vi "PROYECTO.vi"() -> ()   [LabVIEW 2021]
uses:
  <vilib>/userDefined/High Color/IMAQdx.ctl
  <vilib>/addons/database/Connection.llb/DB Tools Open Connec (Path).vi
  <vilib>/Instr/_visa.llb/VISA Configure Serial Port (Instr).vi
  <vilib>/addons/database/Connection.llb/Conn Execute.vi
  <vilib>/addons/database/Recordset.llb/Rec Fetch String Data (R).vi
  <vilib>/addons/database/Recordset.llb/Rec Destroy - Connection.vi
  <vilib>/vision/driver/NI_Vision_Acquisition_Software.lvlib
  <vilib>/vision/NI_Vision_Development_Module.lvlib
  <vilib>/addons/database/NI_Database_API.lvlib
panel:
  in  "VISA resource name":refnum<visa-resource-name>
  in  "connection information":path
  out "Placa Encontrada":string
  out "Consulta":string
  out "Read String":string
  in  "Rectangle":T1 {"Rotation" min=-90.0 max=90.0 step=1.0 format="%.2f"; "Left" scale=0.0..1024.0; "Right" scale=0.0..1024.0}
  out "Image":T2(plugin-control)
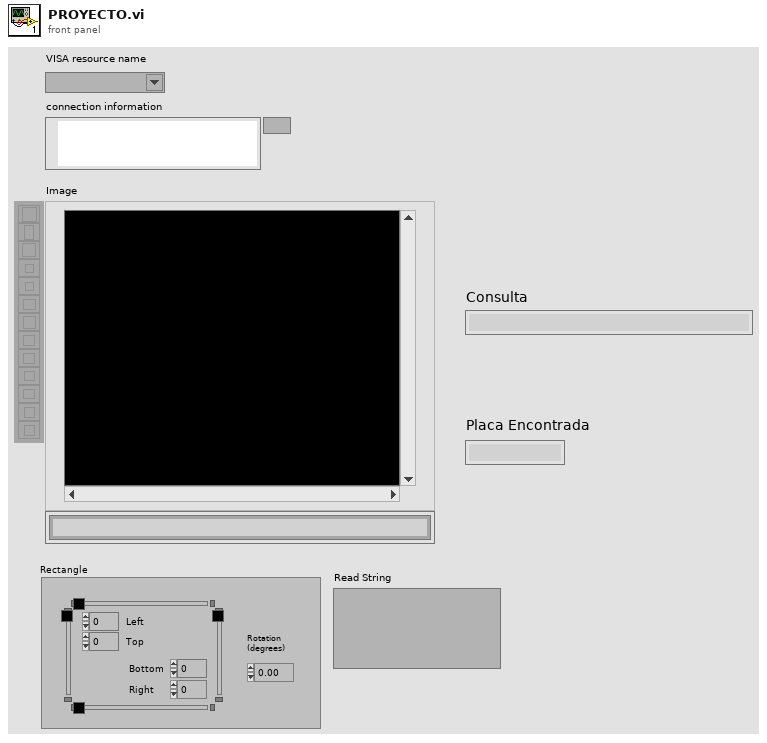
[diagram p1: front panel]
types:
  T1 = typedef "IMAQ Rectangle" = cluster{"Left":i32, "Top":i32, "Right":i32, "Bottom":i32, "Rotation":dbl}
  T2 = typedef "IMAQ Image.ctl" = refnum<image>
  T3 = typedef "IMAQdx.ctl" = refnum<k21>
  T4 = typedef "IMAQ OCR Session.ctl" = refnum<k1>
  T5 = typedef "ROI Descriptor" = cluster{"Global Rectangle":i32[], "Contours":cluster{"ID":enum32{"External", "Internal"}, "Type":u32, "Coordinates":i32[]}[]}
  T6 = typedef "NI_Database_API.lvlib/Conn ObjectReference.ctl" = refnum<k1>
  T7 = cluster{"Global Rectangle":i32[], "Contours":cluster{"ID":enum32{"External", "Internal"}, "Type":u32, "Coordinates":i32[]}[]}
  T8 = typedef "NI_Database_API.lvlib/Rec ObjectReference.ctl" = refnum<k1>
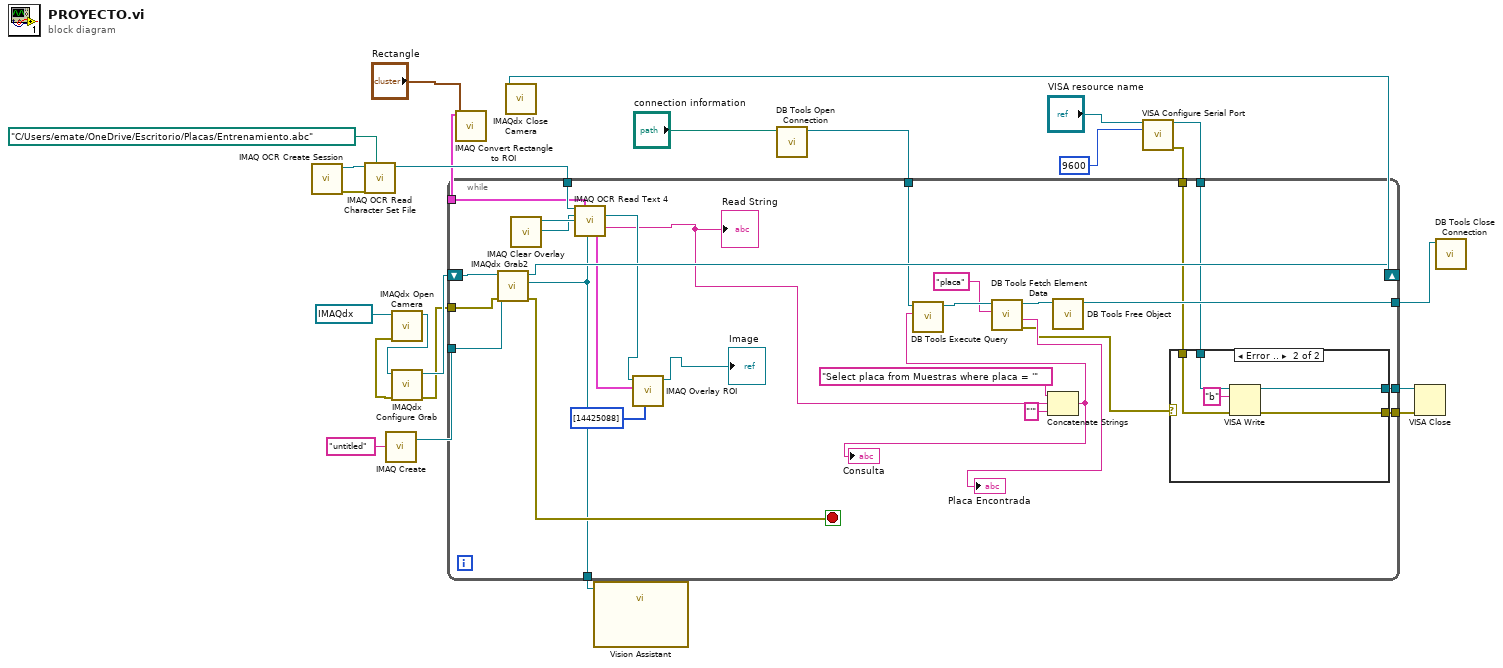
[diagram p0: block diagram]
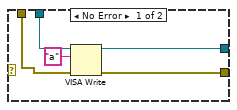
[diagram p2: hidden frame]
diagram:
  n1 = call "IMAQ OCR Create Session"() -> ("error out"=w15:errorcluster, "IMAQ OCR Session"=w16:T4)  [unwired: 10 in]
  n2 = call "IMAQ OCR Read Character Set File"("File Path"=path "C:/Users/emate/OneDrive/Escritorio/Placas/Entrenamiento.abc", "error in (no error)"=w15, "IMAQ OCR Session"=w16) -> ("IMAQ OCR Session (dup)"=w13:T4)  [unwired: 6 in, 2 out]
  n3 = call "IMAQ Create"("Image Name"="untitled") -> ("New Image"=w20:T2)  [unwired: 4 in, 1 out]
  n4 = call <vilib>:"IMAQdx Open Camera.vi"("Session In"=T3 "cam0") -> ("error out"=w23:errorcluster, "Session Out"=w24:T3)  [unwired: 9 in]
  n5 = call <vilib>:"IMAQdx Configure Grab.vi"("error in"=w23, "Session In"=w24) -> ("error out"=w19:errorcluster, "Session Out"=w22:T3)  [unwired: 8 in]
  n6 = call "IMAQ Convert Rectangle to ROI"("Rectangle"="Rectangle") -> ("ROI Descriptor"=w11:T5)  [unwired: 8 in, 1 out]
  n7 = call-poly <vilib>:"DB Tools Open Connection.vi"("connection information"="connection information") -> ("connection reference"=w8:T6)  [unwired: 7 in, 1 out]
  n8 = call-poly "VISA Configure Serial Port"("VISA resource name"="VISA resource name", "baud rate (9600)"=u32 9600) -> ("VISA resource name out"=w4:refnum<visa-resource-name>, "error out"=w3:errorcluster)  [unwired: 12 in]
  n9 = while {
    tunnel: w20 -> [w51]
    tunnel: w19 -> [w50]
    shift-right: [w49] -> w18
    shift-left: w22 -> [w52]
    tunnel: w13 -> [w48]
    tunnel: w11 -> [w47]
    tunnel: [w41] -> w10
    tunnel: w8 -> [w34]
    tunnel: [w29] -> w7
    tunnel: w4 -> [w28]
    tunnel: w3 -> [w27]
    tunnel: [w25] -> w2
    tunnel: [w26] -> w1
    stop <- w46 stop-if-true
    n10 = call <vilib>:"IMAQdx Grab2.vi"("error in"=w50, "Image In"=w51, "Session In"=w52) -> ("error out"=w46:errorcluster, "Image Out"=w41:T2, "Session Out"=w49:T3)  [unwired: 5 in, 1 out]
    n11 = call "IMAQ Clear Overlay"("Image"=w41) -> ("Image Out"=w40:T2)  [unwired: 9 in, 1 out]
    n12 = call "IMAQ OCR Read Text 4"("IMAQ OCR Session"=w48, "ROI Descriptor"=w47, "Image"=w40) -> ("Image (dup)"=w44:T2, "Read String"=w37:string, "ROI Bounding Characters"=w43:T7)  [unwired: 6 in, 4 out]
    "Read String" <- w37
    n13 = call "IMAQ Overlay ROI"("Colors (Green)"=u32[] [14425088], "ROI Descriptor"=w43, "Image"=w44) -> ("Image Out"=→"Image":T2)  [unwired: 7 in, 1 out]
    n14 = Concatenate Strings("Select placa from Muestras where placa = '", w37, "'" ("string")) -> (w33:string)
    "Consulta" <- w33
    n15 = call-poly <vilib>:"DB Tools Execute Query.vi"("SQL query"=w33, "connection reference"=w34) -> ("recordset reference"=w35:T8)  [unwired: 6 in, 1 out]
    n16 = call-poly <vilib>:"DB Tools Fetch Element Data.vi"("column index"="placa", "recordset reference"=w35) -> ("error out"=w30:errorcluster, "data"=→"Placa Encontrada":string, "recordset reference out"=w36:T8)  [unwired: 5 in]
    n17 = call-poly <vilib>:"DB Tools Free Object.vi"("recordset reference"=w36) -> ("connection reference"=w29:T6)  [unwired: 9 in, 1 out]
    n18 = case shown="Error .." w30 {
      tunnel: w28 -> [w55 w62]
      tunnel: w27 -> [w54 w61]
      tunnel: [w56 w58] -> w26
      tunnel: [w57 w59] -> w25
      frame No Error {
        n19 = VISA Write(VISA resource name=w55, write buffer="a", error in (no error)=w54) -> (VISA resource name out=w57:refnum<visa-resource-name>, error out=w56:errorcluster)  [unwired: 1 out]
      }
      frame Error {
        n20 = VISA Write(VISA resource name=w62, write buffer="b", error in (no error)=w61) -> (VISA resource name out=w59:refnum<visa-resource-name>, error out=w58:errorcluster)  [unwired: 1 out]
      }
    }
  }
  n21 = call <vilib>:"IMAQdx Close Camera.vi"("Session In"=w18) -> ()  [unwired: 10 in, 1 out]
  n22 = call "Vision Assistant"("Image In"=w10) -> ()  [unwired: 25 in, 2 out]
  n23 = VISA Close(VISA resource name=w2, error in (no error)=w1) -> ()  [unwired: 1 out]
  n24 = call <vilib>:"DB Tools Close Connection.vi"("connection reference"=w7) -> ()  [unwired: 6 in, 1 out]
